vi "stringToBase64QRCode.vi"(1 "Original":string) -> (0 "Base 64":string)   [LabVIEW 2012]
uses:
  \\vboxsvr\labview-java-example/labview/codecExamples/IKVM.OpenJDK.Core.dll
  IKVM.OpenJDK.Core.dll
  \\VBOXSVR\labview-java-example/SimpleQrExample-DLL/target/Summit.QR.Example.dll
  SimpleQrExample-DLL/target/Summit.QR.Example.dll
panel:
  out "Decoded From Base64 QR":string
  out "Decoded From QR Code":string
  in  "Generate Barcode Button":bool
  out "QR Code":picture
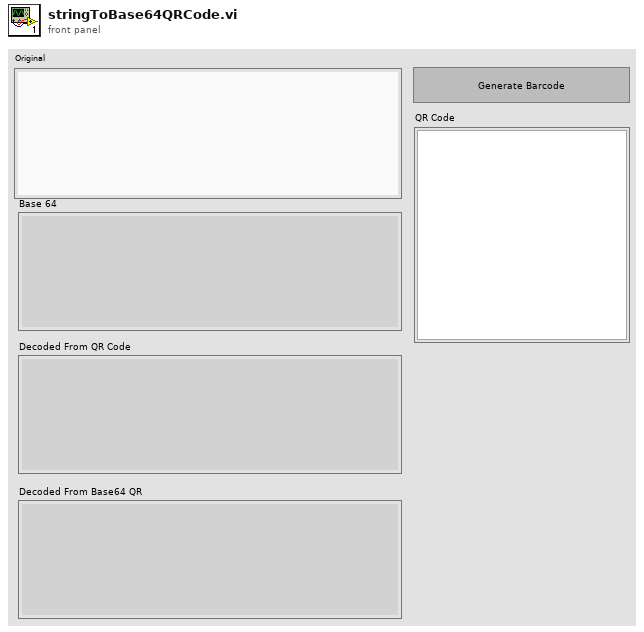
[diagram p1: front panel]
types:
  T1 = typedef "imagedata.ctl" = cluster{"image type":i32, "image depth":i32, "image":u8[], "mask":u8[], "colors":u32[], "Rectangle":cluster{"left":i16, "top":i16, "right":i16, "bottom":i16}}
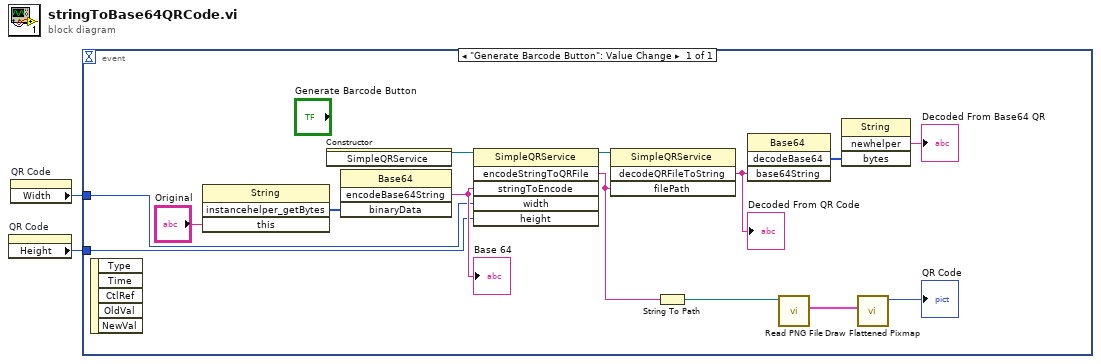
[diagram p0: block diagram]
diagram:
  n1 = property on="QR Code" class="Pict"() -> ("Height"=w1:u32)  [unwired: 2 in, 2 out]
  n2 = property on="QR Code" class="Pict"() -> ("Width"=w2:u32)  [unwired: 2 in, 2 out]
  n3 = event shown="[0] \"Generate Barcode Button\": Value Change" {
    selector: _ -> [_]
    dyn-events: _ -> [_]
    timeout: _ -> [_]
    tunnel: w2 -> [w9]
    tunnel: w1 -> [w8]
    event "Generate Barcode Button": Value Change {
      n4 = event-data() -> ()  [unwired: 1 in, 5 out]
      n5 = invoke class="String" method="instancehelper_getBytes"("this"="Original") -> ("instancehelper_getBytes"=w16:u8[])  [unwired: 3 in, 3 out]
      n6 = constructor class="SimpleQRService"() -> (reference out=w11:refnum<k24>)  [unwired: 3 in, 2 out]
      n7 = invoke class="Base64" method="encodeBase64String"("binaryData"=w16) -> ("encodeBase64String"=w14:string)  [unwired: 3 in, 3 out]
      "Base 64" <- w14
      n8 = invoke class="SimpleQRService" method="encodeStringToQRFile"(reference=w11, "stringToEncode"=w14, "width"=w9, "height"=w8) -> (reference out=w6:refnum<k24>, "encodeStringToQRFile"=w7:string)  [unwired: 2 in, 4 out]
      n9 = invoke class="SimpleQRService" method="decodeQRFileToString"(reference=w6, "filePath"=w7) -> ("decodeQRFileToString"=w5:string)  [unwired: 2 in, 3 out]
      "Decoded From QR Code" <- w5
      n10 = String To Path(string=w7) -> (path=w10:path)
      n11 = invoke class="Base64" method="decodeBase64"("base64String"=w5) -> ("decodeBase64"=w4:u8[])  [unwired: 3 in, 3 out]
      n12 = call <vilib>:"Read PNG File.vi"("path to PNG file"=w10) -> ("image data"=w12:T1)  [unwired: 8 in, 2 out]
      n13 = invoke class="String" method="newhelper"("bytes"=w4) -> ("newhelper"=→"Decoded From Base64 QR":string)  [unwired: 3 in, 3 out]
      n14 = call <vilib>:"Draw Flattened Pixmap.vi"("image data"=w12) -> ("new picture"=→"QR Code":picture)  [unwired: 8 in]
    }
  }
